vi "Channel List to Pins.vi"(0 "Channel List":string) -> (4 "Sites and Pins":string[](array[string]), 6 "Pins":tag[](array[tag]), 8 "Sites":i32[](array[numeric]))   [LabVIEW 2020]
uses:
  <vilib>/Utility/error.llb/whitespace.ctl
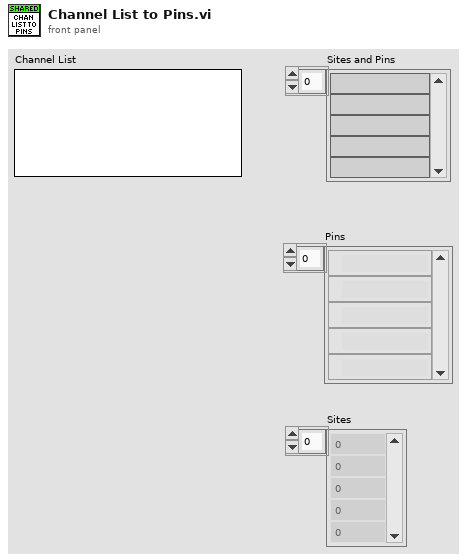
[diagram p1: front panel]
types:
  T1 = typedef "whitespace.ctl" = u16
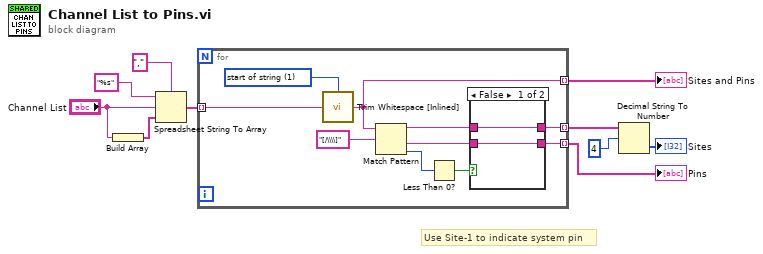
[diagram p0: block diagram]
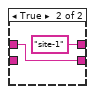
[diagram p2: hidden frame]
diagram:
  # "Use Site-1 to indicate system pin"
  n1 = Build Array("Channel List") -> (w7:string[])
  n2 = Spreadsheet String To Array(delimiter (Tab)=",", format string="%s", spreadsheet string="Channel List", array type (2D Dbl)=w7) -> (array=w6:string[])
  n3 = for {
    tunnel: w6 -> [w20] mode=indexing
    tunnel: [w12] -> w5 mode=indexing
    tunnel: [w11] -> w4 mode=indexing
    tunnel: [w17] -> w3 mode=indexing
    w19 = T1 1 items=["both", "start of string", "end of string"] ("location (both)")
    n4 = call "Trim Whitespace [Inlined].vi"("string"=w20, "location (both)"=w19) -> ("trimmed string"=w17:string)
    n5 = Match Pattern(string=w17, regular expression="[/\\\\]" ("search string/char (-)")) -> (before substring=w13:string, after substring=w14:string, offset past match=w16:i32)  [unwired: 1 in, 1 out]
    n6 = Less Than 0?(x=w16) -> (x < 0?=w15:bool)
    n7 = case shown="False" w15 {
      tunnel: w14 -> [w21 _]
      tunnel: w13 -> [w22 w24]
      tunnel: [w22 "site-1" ("trimmed string")] -> w12
      tunnel: [w21 w24] -> w11
      frame False {
      }
      frame True {
      }
    }
  }
  "Pins" <- w4
  "Sites and Pins" <- w3
  n8 = Decimal String To Number(string=w5, offset=4) -> (number=→"Sites":i32[])  [unwired: 1 in, 1 out]
